vi "Pre Launch Init.vi"(11 "Actor ErrorStop in":refnum<class "Actor ErrorStop.lvclass">) -> (0 "error out":errorcluster, 3 "Actor ErrorStop out":refnum<class "Actor ErrorStop.lvclass">)   [LabVIEW 2012, in "Actor ErrorStop.lvlib" / "Actor ErrorStop.lvclass"]
doc: "(<B>Filename</B>: Actor Framework.lvlib:Actor.lvclass:Pre Launch Init.vi)\n\nDefines behavior that occurs after the Launch Actor method is invoked but before the actor's Actor Core method begins running.\n\nThe Pre Launch Init method is guaranteed to finish before the Launch Actor method returns to its caller and before the actor itself receives any messages. Any references that the Pre Launch Init method obtains are guaranteed to have the same lifetime as the actor itself. Any errors that the Pre Launch Init method returns will abort the launch.\n\nBy default, this method does nothing. A descendant class may override it to define behavior."
uses:
  Actor ErrorStop.lvclass
  <vilib>/ActorFramework/Actor/Actor.lvclass
  Actor ErrorStop.lvclass/Actor ErrorStop.ctl
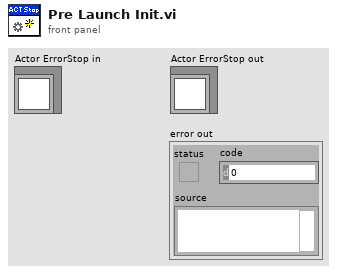
[diagram p1: front panel]
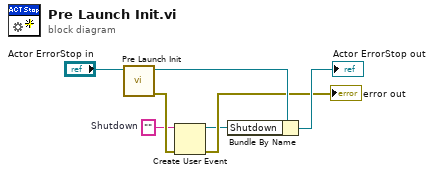
[diagram p0: block diagram]
diagram:
  w2 = ""  # Shutdown
  n1 = call-parent "Pre Launch Init.vi"("Actor in"="Actor ErrorStop in") -> ("error out"=w4:errorcluster, "Actor out"=w6:refnum<class "Actor ErrorStop.lvclass">)  [unwired: 9 in]
  n2 = Create User Event(user event datatype=w2, error in=w4) -> (user event=w1:refnum<user-event>, error out=→"error out":errorcluster)
  n3 = Bundle By Name(cluster=w6, "Shutdown"=w1) -> (→"Actor ErrorStop out":refnum<class "Actor ErrorStop.lvclass">)
